vi "SubConfocal_SetFWpos.vi"(7 "Confocal scanner":T1={"SDC shutter"=FALSE, "Filter wheel"=3, "FW speed"=3, "Disk spinning"=FALSE, "Disk speed (rpm)"=3000.0} {"Disk speed (rpm)" min=1500.0 max=10000.0; "FW speed" min=1 max=5 step=1; "Filter wheel" items=["CFP"=1, "GFP"=2, "mCherry"=3, "Alexa-647"=4, "OFP"=5, "empty"=6]}, 8 "Error In":errorcluster, 11 "Confocal line (VISA IN)":refnum<visa-resource-name>="COM1") -> (0 "Error out":errorcluster, 3 "VISA OUT":refnum<visa-resource-name>)   [LabVIEW 2015]
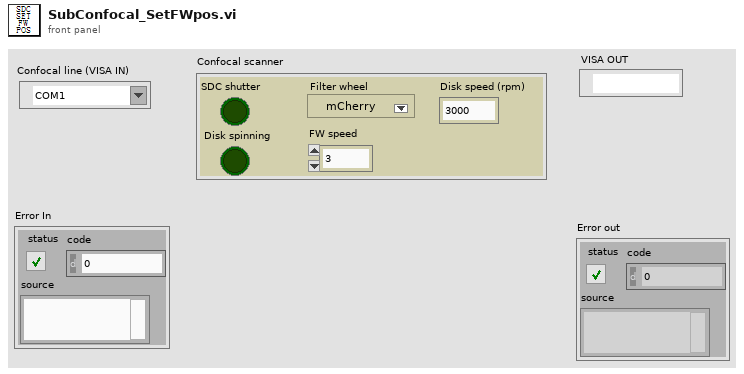
[diagram p1: front panel]
types:
  T1 = cluster{"SDC shutter":bool, "Filter wheel":u16, "FW speed":i32, "Disk spinning":bool, "Disk speed (rpm)":dbl}
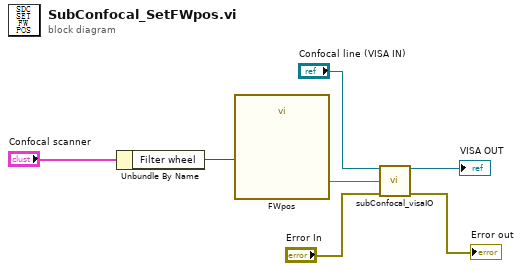
[diagram p0: block diagram]
diagram:
  n1 = Unbundle By Name("Confocal scanner") -> ("Filter wheel"=w1:u16)
  n2 = call "FWpos"("pos"=w1) -> ("Result"=w7:string)  [unwired: 13 in, 1 out]
  n3 = call "subConfocal_visaIO.vi"("VISA  IN"="Confocal line (VISA IN)", "Command (to ctlr)"=w7, "error in"="Error In") -> ("VISA OUT"=→"VISA OUT":refnum<visa-resource-name>, "error out"=→"Error out":errorcluster)  [unwired: 8 in, 3 out]
